vi "Control Indexer.vi"(9 "D-Pad":T3, 10 "Button Cluster":T2, 11 "Axes":T1) -> (3 "Control Label":string)   [LabVIEW 2015]
uses:
  Common Code/Gamepads/D-Pad.ctl
  Common Code/Gamepads/Button Cluster.ctl
  Common Code/Gamepads/Axes Cluster.ctl
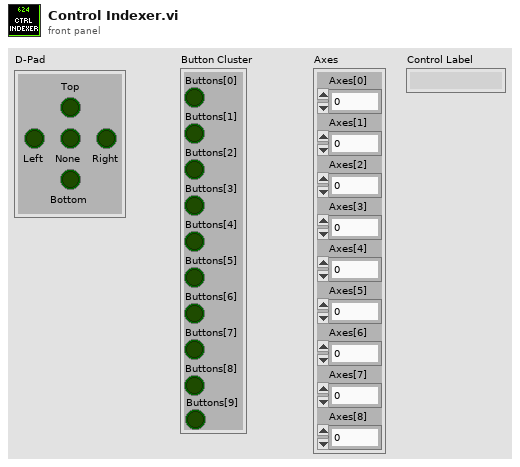
[diagram p1: front panel]
types:
  T1 = typedef "Axes Cluster.ctl" = cluster{"Axes[0]":dbl, "Axes[1]":dbl, "Axes[2]":dbl, "Axes[3]":dbl, "Axes[4]":dbl, "Axes[5]":dbl, "Axes[6]":dbl, "Axes[7]":dbl, "Axes[8]":dbl}
  T2 = typedef "Button Cluster.ctl" = cluster{"Buttons[0]":bool, "Buttons[1]":bool, "Buttons[2]":bool, "Buttons[3]":bool, "Buttons[4]":bool, "Buttons[5]":bool, "Buttons[6]":bool, "Buttons[7]":bool, "Buttons[8]":bool, "Buttons[9]":bool}
  T3 = typedef "D-Pad.ctl" = cluster{"Top":bool, "Bottom":bool, "None":bool, "Right":bool, "Left":bool}
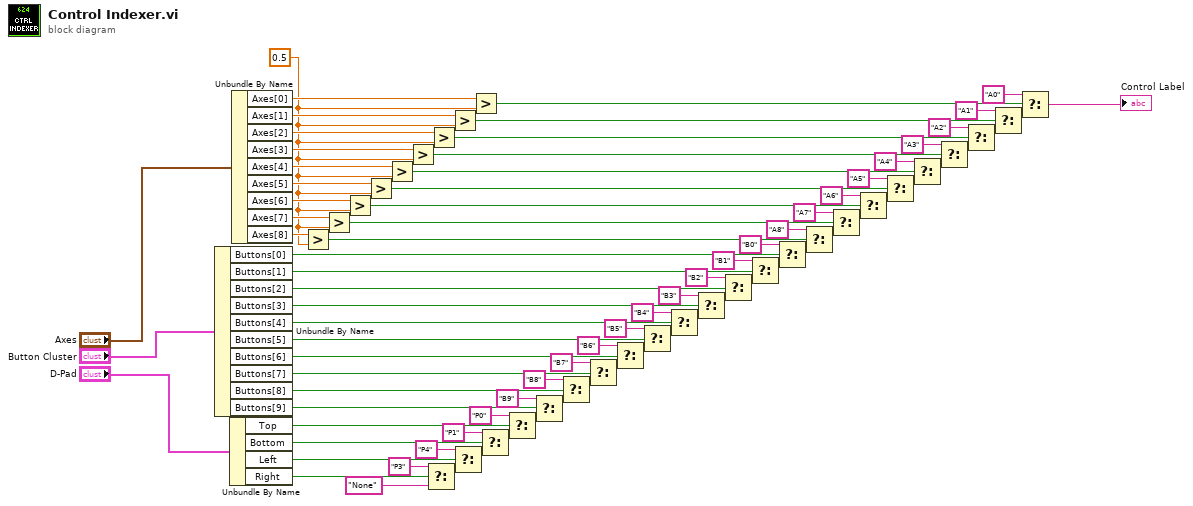
[diagram p0: block diagram]
diagram:
  w74 = 0.5 ("y")
  n1 = Unbundle By Name("Button Cluster") -> ("Buttons[0]"=w57:bool, "Buttons[1]"=w55:bool, "Buttons[2]"=w54:bool, "Buttons[3]"=w53:bool, "Buttons[4]"=w52:bool, "Buttons[5]"=w51:bool, "Buttons[6]"=w50:bool, "Buttons[7]"=w49:bool, "Buttons[8]"=w48:bool, "Buttons[9]"=w46:bool)
  n2 = Unbundle By Name("D-Pad") -> ("Top"=w45:bool, "Bottom"=w44:bool, "Left"=w43:bool, "Right"=w42:bool)
  n3 = Unbundle By Name("Axes") -> ("Axes[0]"=w83:dbl, "Axes[1]"=w82:dbl, "Axes[2]"=w81:dbl, "Axes[3]"=w80:dbl, "Axes[4]"=w79:dbl, "Axes[5]"=w78:dbl, "Axes[6]"=w77:dbl, "Axes[7]"=w76:dbl, "Axes[8]"=w75:dbl)
  n4 = Greater?(x=w75, y=w74) -> (0:w5:bool)
  n5 = Greater?(x=w76, y=w74) -> (0:w6:bool)
  n6 = Greater?(x=w77, y=w74) -> (0:w7:bool)
  n7 = Greater?(x=w78, y=w74) -> (0:w8:bool)
  n8 = Greater?(x=w79, y=w74) -> (0:w9:bool)
  n9 = Greater?(x=w80, y=w74) -> (0:w10:bool)
  n10 = Select(t="P3", s=w42, f="None") -> (s? t:f=w41:string)
  n11 = Greater?(x=w81, y=w74) -> (0:w11:bool)
  n12 = Greater?(x=w82, y=w74) -> (0:w12:bool)
  n13 = Select(t="P4", s=w43, f=w41) -> (s? t:f=w40:string)
  n14 = Greater?(x=w83, y=w74) -> (0:w13:bool)
  n15 = Select(t="P1", s=w44, f=w40) -> (s? t:f=w39:string)
  n16 = Select(t="P0", s=w45, f=w39) -> (s? t:f=w38:string)
  n17 = Select(t="B9", s=w46, f=w38) -> (s? t:f=w47:string)
  n18 = Select(t="B8", s=w48, f=w47) -> (s? t:f=w58:string)
  n19 = Select(t="B7", s=w49, f=w58) -> (s? t:f=w59:string)
  n20 = Select(t="B6", s=w50, f=w59) -> (s? t:f=w60:string)
  n21 = Select(t="B5", s=w51, f=w60) -> (s? t:f=w61:string)
  n22 = Select(t="B4", s=w52, f=w61) -> (s? t:f=w62:string)
  n23 = Select(t="B3", s=w53, f=w62) -> (s? t:f=w63:string)
  n24 = Select(t="B2", s=w54, f=w63) -> (s? t:f=w64:string)
  n25 = Select(t="B1", s=w55, f=w64) -> (s? t:f=w65:string)
  n26 = Select(t="B0", s=w57, f=w65) -> (s? t:f=w56:string)
  n27 = Select(t="A8", s=w5, f=w56) -> (s? t:f=w73:string)
  n28 = Select(t="A7", s=w6, f=w73) -> (s? t:f=w72:string)
  n29 = Select(t="A6", s=w7, f=w72) -> (s? t:f=w71:string)
  n30 = Select(t="A5", s=w8, f=w71) -> (s? t:f=w70:string)
  n31 = Select(t="A4", s=w9, f=w70) -> (s? t:f=w69:string)
  n32 = Select(t="A3", s=w10, f=w69) -> (s? t:f=w68:string)
  n33 = Select(t="A2", s=w11, f=w68) -> (s? t:f=w67:string)
  n34 = Select(t="A1", s=w12, f=w67) -> (s? t:f=w66:string)
  n35 = Select(t="A0", s=w13, f=w66) -> (s? t:f=→"Control Label":string)
